vi "DSF Transfer Group.Move Channels to Engine.vi"(8 "error in (no error)":errorcluster, 11 "Transfer Group in":refnum<class "Transfer Group.lvclass">) -> (0 "error out":errorcluster, 3 "Transfer Group out":refnum<class "Transfer Group.lvclass">)   [LabVIEW 2017, in "DSF.Engine.lvlib" / "Transfer Group.lvclass"]
uses:
  Transfer Group.lvclass
  Transfer Group.lvclass/Transfer Group.ctl
  Transfer.lvclass/Transfer.ctl
  <vilib>/NI/Memory Manager/Classes/Pointer/Memory.Pointer.lvclass/Memory.Pointer.ctl
  <vilib>/NI/Memory Manager/Classes/Pointer/Memory.Pointer.Get Size.vi
  <vilib>/NI/Memory Manager/Classes/Pointer/Memory.Pointer.Copy.vi
  <vilib>/NI/Memory Manager/Classes/Pointer/Memory.Pointer.Copy.No Check.vi
  <vilib>/NI/Memory Manager/Classes/Pointer/Memory.Pointer.Parameter Check.Subset.vi
  <vilib>/NI/Memory Manager/Classes/Pointer/Memory.Pointer.Parameter Check.Null Pointer.vi
  <vilib>/NI/Memory Manager/Classes/Pointer/Memory.Pointer.Get Address.vi
  <vilib>/NI/Memory Manager/Classes/Pointer/Memory.Pointer.Errors.vi
  <vilib>/NI/Memory Manager/Classes/Pointer/Memory.Pointer.Errors.Out of Bounds.vi
  <vilib>/NI/Memory Manager/Classes/Pointer/Memory.Pointer.Errors.Null Pointer.vi
  <vilib>/NI/Memory Manager/VIs/Source.Write.String.vi
  <vilib>/NI/Memory Manager/Classes/Pointer/Memory.Pointer.Errors.Write Pointer Size.vi
  <vilib>/NI/Memory Manager/Classes/Pointer/Memory.Pointer.Errors.Create Error.vi
  <vilib>/NI/Memory Manager/VIs/Source.Write.Scalar.Base10.vi
  <vilib>/NI/Memory Manager/VIs/Source.Write.Scalar.Base10 (U64).vi
  <vilib>/NI/Memory Manager/VIs/New Error Cluster Constant.vi
  <vilib>/NI/Memory Manager/VIs/New Error Cluster Constant (512B).vi
  <vilib>/NI/Memory Manager/VIs/Error Cluster.Set Status.vi
  <vilib>/NI/Memory Manager/VIs/Error Cluster.Set Code.vi
  <vilib>/NI/Memory Manager/VIs/Error Cluster.Set VI Source.vi
  <vilib>/NI/Memory Manager/Constants/Memory.Constants.vi
  <vilib>/NI/Memory Manager/Constants/Memory.Constants.Library Name.vi
  <vilib>/NI/Memory Manager/Classes/Pointer/Memory.Pointer.Errors.Get Info.vi
  Pointer/DBL Pointer.lvclass
  C:/Program Files (x86)/National Instruments/LabVIEW 2017/vi.lib/NI/Memory Manager/Classes/Pointer/Memory.Pointer.lvclass
  Transfer.lvclass
  <vilib>/NI/Memory Manager/Classes/Pointer/Memory.Pointer.lvclass
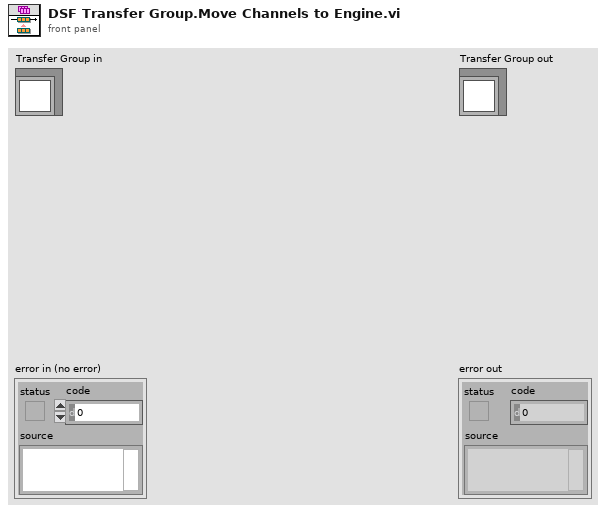
[diagram p1: front panel]
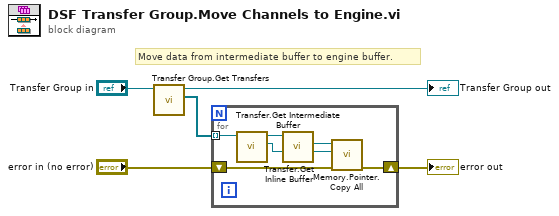
[diagram p0: block diagram]
diagram:
  # "Move data from intermediate buffer to engine buffer."
  n1 = call "Transfer Group.Get Transfers.vi"("Transfer Group in"="Transfer Group in") -> ("Transfers"=w4:refnum<class "Transfer.lvclass">[], "Transfer Group out"=→"Transfer Group out":refnum<class "Transfer Group.lvclass">)  [unwired: 9 in]
  n2 = for {
    tunnel: w4 -> [w9] mode=indexing
    shift-right: [w11] -> w2
    shift-left: "error in (no error)" -> [w10]
    n3 = call "Transfer.Get Intermediate Buffer.vi"("Transfer in"=w9) -> ("DBL Buffer"=w8:refnum<class "DBL Pointer.lvclass">, "Transfer out"=w7:refnum<class "Transfer.lvclass">)  [unwired: 9 in]
    n4 = call "Transfer.Get Inline Buffer.vi"("Transfer in"=w7) -> ("Inline Buffer"=w6:refnum<class "DBL Pointer.lvclass">)  [unwired: 9 in, 1 out]
    n5 = call <vilib>:"Memory.Pointer.Copy All.vi"("error in (no error)"=w10, "dst Pointer in"=w8, "src Pointer in"=w6) -> ("error out"=w11:errorcluster)  [unwired: 6 in, 2 out]
  }
  "error out" <- w2
